vi "Title (SubVI).vi"(11 "About_prg":T1) -> (3 "String":string)   [LabVIEW 2017]
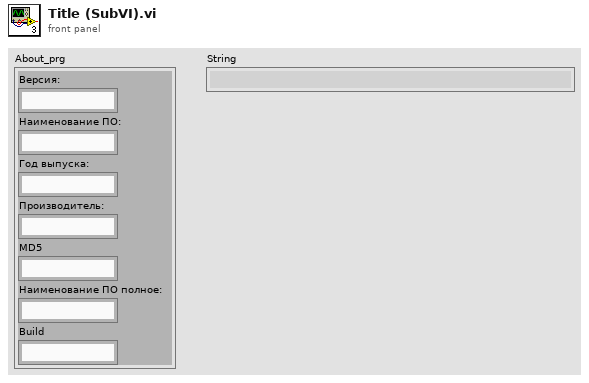
[diagram p1: front panel]
types:
  T1 = cluster{"Версия:":string, "Наименование ПО:":string, "Год выпуска:":string, "Производитель:":string, "MD5":string, "Наименование ПО полное:":string, "Build":string}
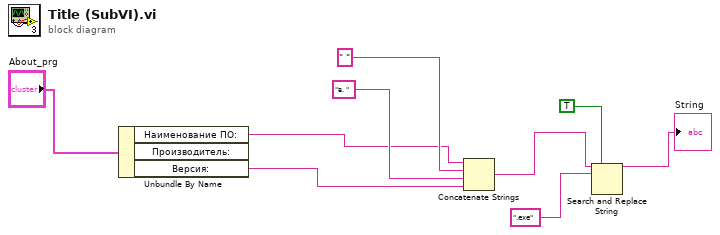
[diagram p0: block diagram]
diagram:
  n1 = Unbundle By Name("About_prg") -> ("Наименование ПО:"=w5:string, "Версия:"=w9:string)  [unwired: 1 out]
  n2 = Concatenate Strings(w5, " " ("string"), "в. " ("string"), w9) -> (w4:string)
  n3 = Search and Replace String(replace all?=TRUE ("replace all? (F)"), input string=w4, search string=".exe") -> (result string=→"String":string)  [unwired: 5 in, 3 out]
